vi "Check ROI Type (Closed or Open).vi"(8 "Error In":errorcluster, 11 "ROI Descriptor":T1 {"Contours"."Type" items=["No Selection", "Point", "Line", "Rectangle", "Oval", "Polygon", "Freehand Region", "Annulus", "Unused2", "Unused3", "Broken Line", "Freehand Line", "Rotated Rectangle"]}) -> (0 "Error Out":errorcluster, 1 "Closed ROI":bool, 2 "Curve":bool, 3 "ROI Descriptor dup":T1 {"Contours"."Type" items=["No Selection", "Point", "Line", "Rectangle", "Oval", "Polygon", "Freehand Region", "Annulus", "Unused2", "Unused3", "Broken Line", "Freehand Line", "Rotated Rectangle"]}, 4 "Array of points":bool)   [LabVIEW 2021, in "Image.lvlib"]
uses:
  Image.lvlib
  Image ROI Type.ctl
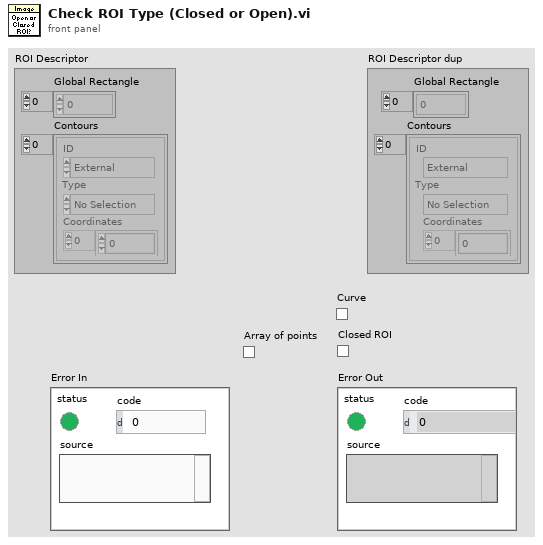
[diagram p1: front panel]
types:
  T1 = typedef "ROI Descriptor" = cluster{"Global Rectangle":i32[], "Contours":cluster{"ID":enum32{"External", "Internal"}, "Type":u32, "Coordinates":i32[]}[]}
  T2 = typedef "Image.lvlib/Image ROI Type.ctl" = enum16{"No Selection", "Point", "Line", "Rectangle", "Oval", "Polygon", "Freehand Region", "Annulus", "Unused2", "Unused3", "Broken Line", "Freehand Line", "Rotated Rectangle"}
  T3 = cluster{"ID":enum32{"External", "Internal"}, "Type":u32, "Coordinates":i32[]}[]
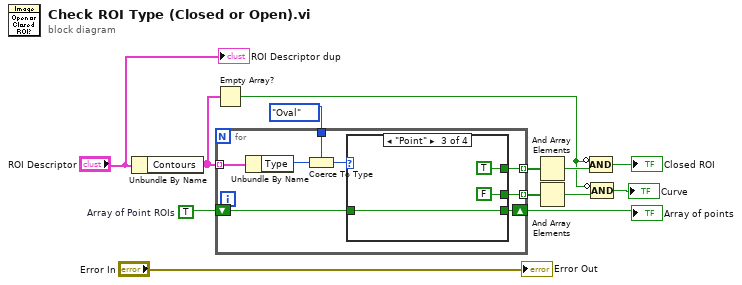
[diagram p0: block diagram]
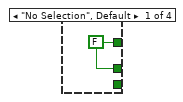
[diagram p2: hidden frame]
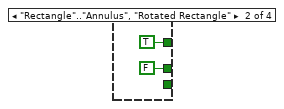
[diagram p3: hidden frame]
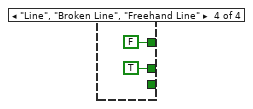
[diagram p4: hidden frame]
diagram:
  w2 = TRUE  # Array of Point ROIs
  n1 = Unbundle By Name("ROI Descriptor") -> ("Contours"=w6:T3)
  n2 = Empty Array?(array=w6) -> (empty?=w3:bool)
  n3 = for {
    tunnel: w6 -> [w21] mode=indexing
    tunnel: Image_ROI_Type."Oval" ("ROI Type") -> [w19]
    tunnel: [w17] -> w10 mode=indexing
    tunnel: [w16] -> w9 mode=indexing
    shift-right: [w14] -> w1
    shift-left: w2 -> [w15]
    n4 = Unbundle By Name(w21) -> ("Type"=w20:u32)
    n5 = Coerce To Type(0:w20, 1:w19) -> (2:w18:T2)
    n6 = case shown="\"Point\"" w18 {
      tunnel: [w22 TRUE ("Valid Profile ROI") TRUE ("Valid Profile ROI") FALSE ("Valid Profile ROI")] -> w17
      tunnel: [w22 FALSE ("Valid Profile ROI") FALSE ("Valid Profile ROI") TRUE ("Valid Profile ROI")] -> w16
      tunnel: w15 -> [_ _ w25 _]
      tunnel: [_ _ w25 _] -> w14
      frame "No Selection", Default {
        w22 = FALSE ("Valid Profile ROI")
      }
      frame "Rectangle".."Annulus", "Rotated Rectangle" {
      }
      frame "Point" {
      }
      frame "Line", "Broken Line", "Freehand Line" {
      }
    }
  }
  "Array of points" <- w1
  n7 = And Array Elements(Boolean array=w10) -> (logical AND=w8:bool)
  n8 = And Array Elements(Boolean array=w9) -> (logical AND=w7:bool)
  n9 = Compound Arithmetic op=AND(invert w3, w8) -> (→"Closed ROI":bool)
  n10 = Compound Arithmetic op=AND(invert w3, w7) -> (→"Curve":bool)
  "ROI Descriptor dup" <- "ROI Descriptor"
  "Error Out" <- "Error In"
